vi "WS1050 Bench CAP Characterization_Ver1.3.vi"() -> ()   [LabVIEW 2012]
panel:
  in  "Cmd Full":string[](array[string])=["00", "01", "02", "03", "04", "05", "06", "07", "08", "09", "0A", "0B", "0C", "0D", "0E", "0F", "10", "11", "12", "13", "14", "15", "16", "17", "18", "19", "1A", "1B", "1C", "1D", "1E", "1F", "20", "21", "22", "23", "24", "25", "26", "27", "28", "29", "2A", "2B", "2C", "2D", "2E", "2F", "30", "31", "32", "33", "34", "35", "36", "37", "38", "39", "3A", "3B", "3A", "39", "38", "37", "36", "35", "34", "33", "32", "31", "30", "2F", "2E", "2D", "2C", "2B", "2A", "29", "28", "27", "26", "25", "24", "23", "22", "21", "20", "1F", "1E", "1D", "1C", "1B", "1A", "19", "18", "17", "16", "15", "14", "13", "12", "11", "10", "0F", "0E", "0D", "0C", "0B", "0A", "09", "08", "07", "06", "05", "04", "03", "02", "01", "00"]
  in  "Driver Name Full":string[](array[string])=["C1_Min", "F1_UP", "F2_UP", "F12_UP", "S1_UP", "S1F1_UP", "S1F2_UP", "S1F12_UP", "S2_UP", "S2F1_UP", "S2F2_UP", "S2F12_UP", "S3_UP", "S3F1_UP", "S3F2_UP", "S3F12_UP", "S4_UP", "S4F1_UP", "S4F2_UP", "S4F12_UP", "S5_UP", "S5F1_UP", "S5F2_UP", "S5F12_UP", "S6_UP", "S6F1_UP", "S6F2_UP", "S6F12_UP", "S7_UP", "S7F1_UP", "S7F2_UP", "S7F12_UP", "S8_UP", "S8F1_UP", "S8F2_UP", "S8F12_UP", "S9_UP", "S9F1_UP", "S9F2_UP", "S9F12_UP", "S10_UP", "S10F1_UP", "S10F2_UP", "S10F12_UP", "S11_UP", "S11F1_UP", "S11F2_UP", "S11F12_UP", "S12_UP", "S12F1_UP", "S12F2_UP", "S12F12_UP", "S13_UP", "S13F1_UP", "S13F2_UP", "S13F12_UP", "S14_UP", "S14F1_UP", "S14F2_UP", "S14F12_UP", "S14F2_DN", "S14F1_DN", "S14_DN", "S13F12_DN", "S13F2_DN", "S13F1_DN", "S13_DN", "S12F12_DN", "S12F2_DN", "S12F1_DN", "S12_DN", "S11F12_DN", "S11F2_DN", "S11F1_DN", "S11_DN", "S10F12_DN", "S10F2_DN", "S10F1_DN", "S10_DN", "S9F12_DN", "S9F2_DN", "S9F1_DN", "S9_DN", "S8F12_DN", "S8F2_DN", "S8F1_DN", "S8_DN", "S7F12_DN", "S7F2_DN", "S7F1_DN", "S7_DN", "S6F12_DN", "S6F2_DN", "S6F1_DN", "S6_DN", "S5F12_DN", "S5F2_DN", "S5F1_DN", "S5_DN", "S4F12_DN", "S4F2_DN", "S4F1_DN", "S4_DN", "S3F12_DN", "S3F2_DN", "S3F1_DN", "S3_DN", "S2F12_DN", "S2F2_DN", "S2F1_DN", "S2_DN", "S1F12_DN", "S1F2_DN", "S1F1_DN", "S1_DN", "F12_DN", "F2_DN", "F1_DN", "ALL_OFF"]
  in  "Tab Control":enum32{"CONTROL", "INDICATION"}(tab)
  in  "RFFE Com Port":refnum<visa-resource-name>="COM3"
  in  "AD7747 Com Port":refnum<visa-resource-name>="COM1"
  in  "Init":bool=TRUE
  in  "Wafer":string="WS1050"
  in  "Lot":string="Toggle 7"
  in  "SN":string="01"
  in  "Temperature":string="RT"
  in  "Delay(ms)":u32=100
  in  "TMN DC\\CAP Data Log File Path":path=path "C:/Andy Tr/Temp"
  in  "String":string="WS1050 BENCH CAP CHARACTERIZATION Ver1.3"
  out "C3Cal (pF)":dbl=-4.9974111328125
  out "C1Cal (pF)":dbl=-4.5642919921875
  out "C2Cal (pF)":dbl=-4.9191376953125
  out "S_ValueC3(pF)":dbl=-4.9974111328125
  out "S_ValueC1(pF)":dbl=-4.5642919921875
  out "S_ValueC2(pF)":dbl=-4.9191376953125
  in  "Calib Socket":bool
  out "C1_Mesa(pF)":dbl
  out "C2_Mesa(pF)":dbl
  out "C3_Mesa(pF)":dbl
  in  "A364X_VDD":refnum<visa-resource-name>="GPIB1::6::INSTR"
  in  "IDD Limit":dbl=0.02 format="%.2p"
  in  "VDD":dbl=3.3
  in  "CP Setting":i32(ring) items=["CP OFF", "CP ON", "DVA OFF", "DVA ON", "ECAL OFF", "ECAL ON", "CP 40.25V", "CP 35V", "CP 38V", "CP 44V", "CP 50V", "CP 23.75V", "CP 25.25V", "CP 29.75V", "C1 ON", "C1 OFF", "C2 ON", "C2 OFF", "C3 ON", "C3 OFF"]
  in  "Send":bool
  in  "Init AD7747":bool
  in  "Keithley 2000":refnum<visa-resource-name>
  out "C_min(pF)":string[](array[string])
  out "C_Max":string[](array[string])
  out "C_Min2(pF)":string[](array[string])
  out "error out":errorcluster
  in  "error in (no error)":errorcluster
  in  "stop":bool
  in  "Abort":bool
  in  "Start Test":bool
  out "Running loop":i32
  in  "Set Cmax":string[](array[string])=["07413B", "07423B", "07433B"]
  out "CMin_Hex":string[](array[string])
  out "CMax_Hex":string[](array[string])
  out "CMin2 Hex":string[](array[string])
  # "Company:  WiSpry Inc\n198 Fairbanks Ste 198 Irvine\n\nCreated by:  Andy V Tran\nDate:  03/11/2015\nTP:  WS1050 Bench\nCAP Characterization"
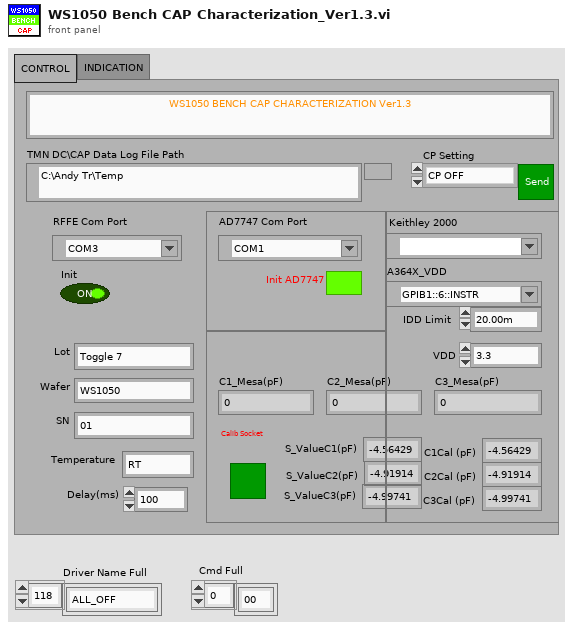
[diagram p1: front panel]
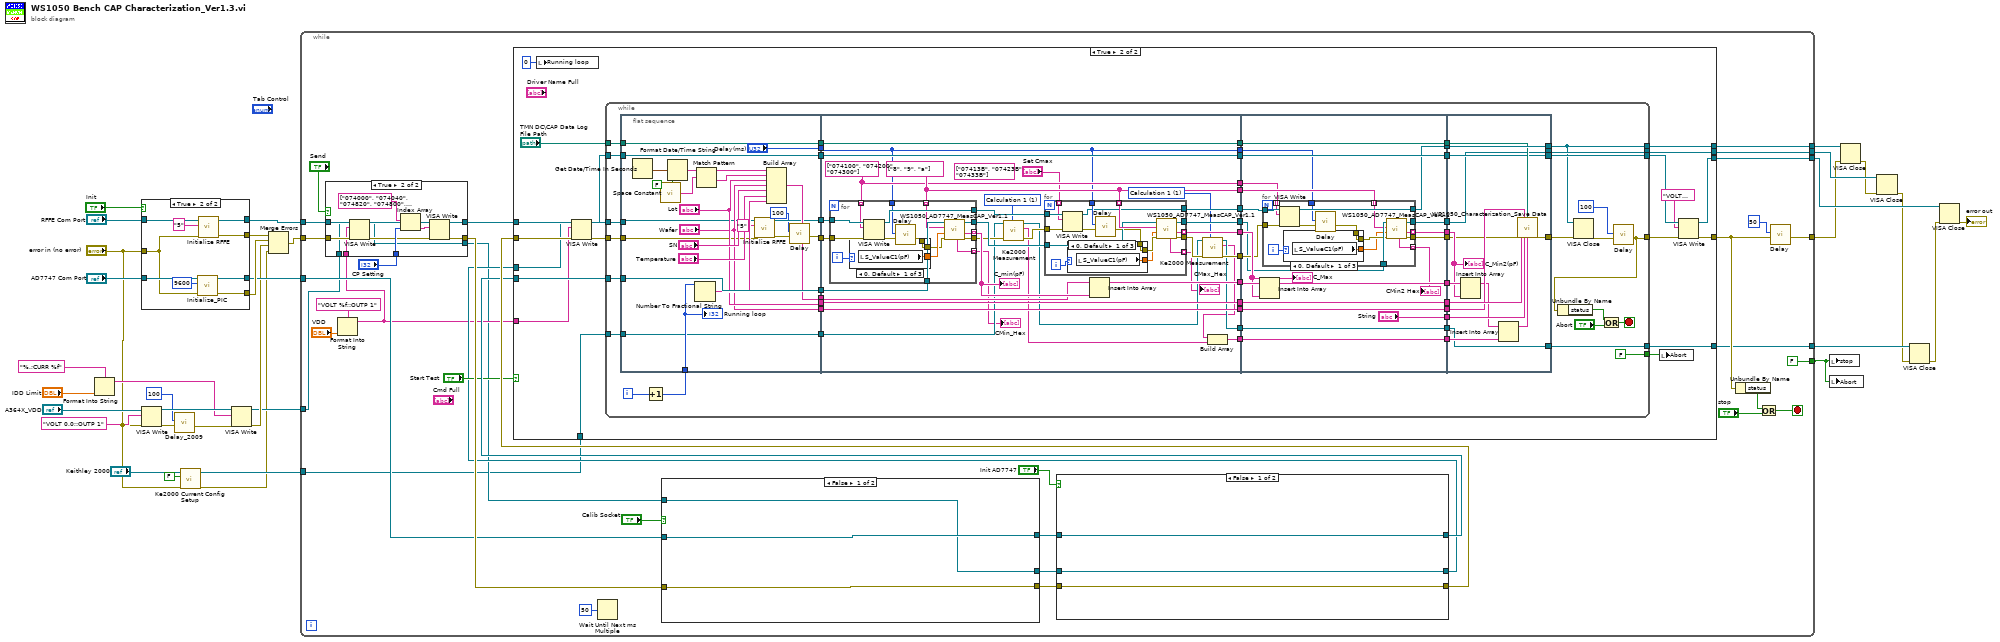
[diagram p0: block diagram]
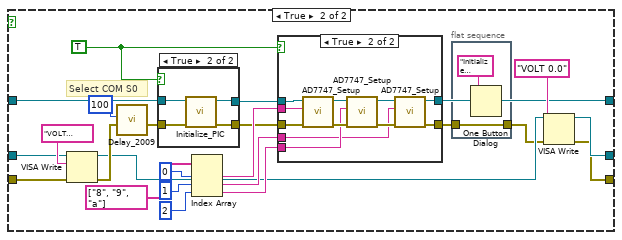
[diagram p3: hidden frame]
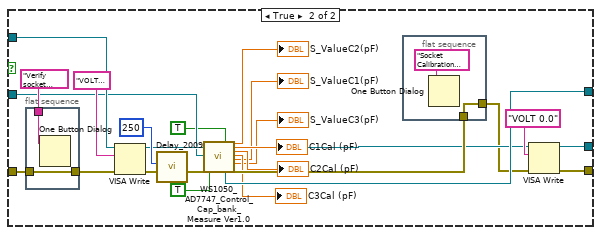
[diagram p6: hidden frame]
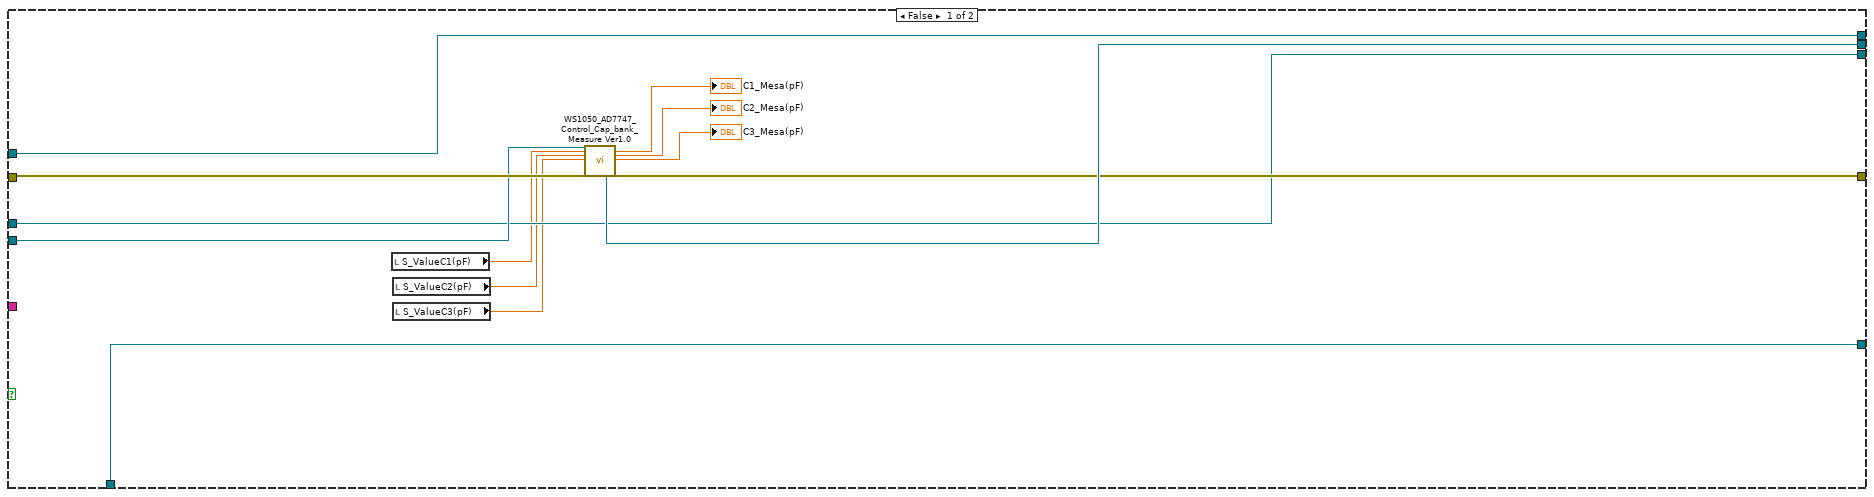
[diagram p7: hidden frame]
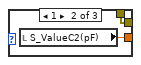
[diagram p8: hidden frame]
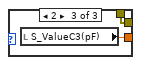
[diagram p9: hidden frame]
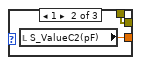
[diagram p10: hidden frame]
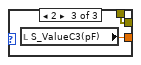
[diagram p11: hidden frame]
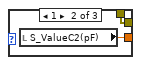
[diagram p12: hidden frame]
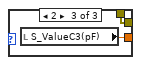
[diagram p13: hidden frame]
diagram:
  n1 = Format Into String(format string="%.;CURR %f", "IDD Limit") -> (resulting string=w24:string)  [unwired: 2 in, 1 out]
  n2 = case shown="True" "Init" {
    tunnel: "RFFE Com Port" -> [w37 w46]
    tunnel: [w37 w44] -> w33
    tunnel: "AD7747 Com Port" -> [w35 w42]
    tunnel: [w36 w41] -> w31
    tunnel: [w36 w40] -> w30
    tunnel: [w35 w39] -> w28
    tunnel: "error in (no error)" -> [w36 w38]
    frame False {
    }
    frame True {
      n3 = call "Initialize_PIC.vi"("error in (no error)"=w38, "baud rate"=u32 9600, "Select Com Port"=w42) -> ("error out"=w40:errorcluster, "VISA resource name out"=w39:refnum<visa-resource-name>)  [unwired: 7 in]
      n4 = call "Initialize RFFE.vi"("error in (no error)"=w38, "write buffer"="5", "Select Com Port"=w46) -> ("error out"=w41:errorcluster, "VISA resource name out"=w44:refnum<visa-resource-name>)  [unwired: 7 in]
    }
  }
  n5 = VISA Write(VISA resource name="A364X_VDD", write buffer="VOLT 0.0;:OUTP 1", error in (no error)="error in (no error)") -> (VISA resource name out=w25:refnum<visa-resource-name>, error out=w21:errorcluster)  [unwired: 1 out]
  n6 = call "Delay_2009.vi"("error in (no error)"=w21, "milliseconds to wait"=u32 100) -> ("error out"=w26:errorcluster)  [unwired: 9 in]
  n7 = call "Ke2000 Current Config Setup.vi"("error in (no error)"="error in (no error)", "Auto Range(T/F)"=FALSE, "VISA resource name"="Keithley 2000") -> ("error out"=w4:errorcluster, "VISA resource name out"=w5:refnum<visa-resource-name>)  [unwired: 7 in]
  n8 = VISA Write(VISA resource name=w25, write buffer=w24, error in (no error)=w26) -> (VISA resource name out=w16:refnum<visa-resource-name>, error out=w17:errorcluster)  [unwired: 1 out]
  n9 = Merge Errors(w31, w30, w17, w4) -> (w29:errorcluster)
  n10 = while {
    tunnel: w33 -> [w77]
    tunnel: w29 -> [w78]
    tunnel: w28 -> [w65]
    tunnel: [w73] -> w12
    tunnel: [w71] -> w15
    tunnel: [w70] -> w14
    tunnel: w16 -> [w52]
    tunnel: [w56] -> w13
    tunnel: [FALSE ("stop")] -> w9
    tunnel: w5 -> [w48]
    tunnel: [w47] -> w3
    stop <- w68 stop-if-true
    n11 = Format Into String(format string="VOLT %f;:OUTP 1", "VDD") -> (resulting string=w51:string)  [unwired: 2 in, 1 out]
    n12 = case shown="True" "Send" {
      tunnel: w78 -> [w410 w416]
      tunnel: [w410 w420] -> w66
      tunnel: [w409 w419] -> w76
      tunnel: "CP Setting" -> [_ w418]
      tunnel: w77 -> [w409 w417]
      tunnel: w52 -> [w408 w415]
      tunnel: w51 -> [_ w414]
      tunnel: [w408 w412] -> w50
      frame False {
      }
      frame True {
        n13 = VISA Write(VISA resource name=w415, write buffer=w414, error in (no error)=w416) -> (VISA resource name out=w412:refnum<visa-resource-name>, error out=w413:errorcluster)  [unwired: 1 out]
        n14 = Index Array(array=string[] ["074000", "074040", "074820", "074800", "074044", "074040", "074776", "07476F", "074773", "07477B", "07477C", "074760", "074762", "074768", "07413B", "074100", "07423B", "074200", "07433B", "074300"], index=w418) -> (element=w421:string)
        n15 = VISA Write(VISA resource name=w417, write buffer=w421, error in (no error)=w413) -> (VISA resource name out=w419:refnum<visa-resource-name>, error out=w420:errorcluster)  [unwired: 1 out]
      }
    }
    n16 = Wait Until Next ms Multiple(millisecond multiple=u32 50) -> ()  [unwired: 1 out]
    n17 = case shown="False" "Calib Socket" {
      tunnel: w66 -> [w131 w154]
      tunnel: [w131 w137] -> w60
      tunnel: w65 -> [w130 w135]
      tunnel: w50 -> [w129 w143]
      tunnel: [w129 w138] -> w61
      tunnel: [w130 w152] -> w59
      frame False {
      }
      frame True {
        n18 = flat-sequence {
          tunnel: [w157] -> w144
          tunnel: w154 -> [w157]
          tunnel: "Verify socket should be empty" ("message") -> [w156]
          frame #0 {
            n19 = One Button Dialog(message=w156) -> ()  [unwired: 1 in, 1 out]
          }
        }
        n20 = VISA Write(VISA resource name=w143, write buffer="VOLT 3.3;:OUTP 1", error in (no error)=w144) -> (VISA resource name out=w139:refnum<visa-resource-name>, error out=w141:errorcluster)  [unwired: 1 out]
        n21 = call "Delay_2009.vi"("error in (no error)"=w141, "milliseconds to wait"=u32 250) -> ("error out"=w134:errorcluster)  [unwired: 9 in]
        n22 = call "WS1050_AD7747_Control_Cap_bank_Measure Ver1.0.vi"("Select Com Port"=w135, "errorin"=w134, "Push Button to Measue Cap"=TRUE, "Push Button to Calibrate"=TRUE ("Push Button to Initialize AD7747")) -> ("Com Port Out"=w152:refnum<visa-resource-name>, "C2(pF)"=→"S_ValueC2(pF)":dbl, "C1_Mesa(pF)"=→"C1Cal (pF)":dbl, "C2_Mesa(pF)"=→"C2Cal (pF)":dbl, "C3_Mesa(pF)"=→"C3Cal (pF)":dbl, "C1(pF)"=→"S_ValueC1(pF)":dbl, "C3(pF)"=→"S_ValueC3(pF)":dbl, "error out"=w153:errorcluster)  [unwired: 16 in]
        n23 = flat-sequence {
          tunnel: [w158] -> w136
          tunnel: w153 -> [w158]
          frame #0 {
            n24 = One Button Dialog(message="Socket Calibration Completed, Please insert DUT into the Socket") -> ()  [unwired: 1 in, 1 out]
          }
        }
        n25 = VISA Write(VISA resource name=w139, write buffer="VOLT 0.0", error in (no error)=w136) -> (VISA resource name out=w138:refnum<visa-resource-name>, error out=w137:errorcluster)  [unwired: 1 out]
      }
    }
    n26 = case shown="False" "Init AD7747" {
      tunnel: w59 -> [w82 w107]
      tunnel: [w83 w87] -> w63
      tunnel: w60 -> [w83 w92]
      tunnel: [w82 w85] -> w62
      tunnel: w61 -> [w81 w93]
      tunnel: [w81 w88] -> w57
      frame False {
      }
      frame True {
        w97 = TRUE
        # "Select COM S0"
        n27 = VISA Write(VISA resource name=w93, write buffer="VOLT 3.3;:OUTP 1", error in (no error)=w92) -> (VISA resource name out=w89:refnum<visa-resource-name>, error out=w91:errorcluster)  [unwired: 1 out]
        n28 = call "Delay_2009.vi"("error in (no error)"=w91, "milliseconds to wait"=u32 100) -> ("error out"=w95:errorcluster)  [unwired: 9 in]
        n29 = case shown="True" w97 {
          tunnel: [w121 w126] -> w98
          tunnel: [w122 w125] -> w106
          tunnel: w107 -> [w122 w124]
          tunnel: w95 -> [w121 w123]
          frame False {
          }
          frame True {
            n30 = call "Initialize_PIC.vi"("error in (no error)"=w123, "Select Com Port"=w124) -> ("error out"=w126:errorcluster, "VISA resource name out"=w125:refnum<visa-resource-name>)  [unwired: 8 in]
          }
        }
        n31 = Index Array(array=string[] ["8", "9", "a"], index #1=0 ("index"), index #2=1 ("index"), index #3=2 ("index")) -> (element #1=w101:string, element #2=w100:string, element #3=w99:string)
        n32 = case shown="True" w97 {
          tunnel: w98 -> [w109 w112]
          tunnel: [w109 w110] -> w84
          tunnel: w106 -> [w108 w120]
          tunnel: w101 -> [_ w115]
          tunnel: w99 -> [_ w114]
          tunnel: w100 -> [_ w113]
          tunnel: [w108 w111] -> w85
          frame False {
          }
          frame True {
            n33 = call "AD7747_Setup.vi"("error in"=w112, "AD7747_Number"=w115, "Control"=w120) -> ("error out"=w119:errorcluster, "Control out"=w118:refnum<visa-resource-name>)  [unwired: 6 in, 1 out]
            n34 = call "AD7747_Setup.vi"("error in"=w119, "AD7747_Number"=w114, "Control"=w118) -> ("error out"=w117:errorcluster, "Control out"=w116:refnum<visa-resource-name>)  [unwired: 6 in, 1 out]
            n35 = call "AD7747_Setup.vi"("error in"=w117, "AD7747_Number"=w113, "Control"=w116) -> ("error out"=w110:errorcluster, "Control out"=w111:refnum<visa-resource-name>)  [unwired: 6 in, 1 out]
          }
        }
        n36 = flat-sequence {
          tunnel: w84 -> [w127]
          tunnel: [w127] -> w86
          frame #0 {
            n37 = One Button Dialog(message="Initialize AD7747 completed!") -> ()  [unwired: 1 in, 1 out]
          }
        }
        n38 = VISA Write(VISA resource name=w89, write buffer="VOLT 0.0", error in (no error)=w86) -> (VISA resource name out=w88:refnum<visa-resource-name>, error out=w87:errorcluster)  [unwired: 1 out]
      }
    }
    n39 = case shown="True" "Start Test" {
      tunnel: w76 -> [w165 w191]
      tunnel: w63 -> [w172 w186]
      tunnel: w62 -> [w171 w190]
      tunnel: [w169 w184] -> w74
      tunnel: [w165 w189] -> w71
      tunnel: [w170 w188] -> w70
      tunnel: w57 -> [w164 w185]
      tunnel: [w164 w181] -> w56
      tunnel: w51 -> [_ w176]
      tunnel: w48 -> [w160 w174]
      tunnel: [w160 w173] -> w47
      frame False {
        n40 = local read "S_ValueC1(pF)"() -> (w163:dbl)
        n41 = local read "S_ValueC2(pF)"() -> (w162:dbl)
        n42 = local read "S_ValueC3(pF)"() -> (w161:dbl)
        n43 = call "WS1050_AD7747_Control_Cap_bank_Measure Ver1.0.vi"("Select Com Port"=w171, "S_Value C1"=w163, "S_Value C2"=w162, "S_Value C3"=w161, "errorin"=w172) -> ("Com Port Out"=w170:refnum<visa-resource-name>, "C1_Mesa(pF)"=→"C1_Mesa(pF)":dbl, "C2_Mesa(pF)"=→"C2_Mesa(pF)":dbl, "C3_Mesa(pF)"=→"C3_Mesa(pF)":dbl, "error out"=w169:errorcluster)  [unwired: 15 in, 3 out]
      }
      frame True {
        n44 = local write "Running loop"(0 ("Loop Running")) -> ()
        n45 = VISA Write(VISA resource name=w185, write buffer=w176, error in (no error)=w186) -> (VISA resource name out=w183:refnum<visa-resource-name>, error out=w187:errorcluster)  [unwired: 1 out]
        n46 = while {
          tunnel: w191 -> [w244]
          tunnel: w187 -> [w243]
          tunnel: w190 -> [w242]
          tunnel: [w192] -> w180
          tunnel: "TMN DC\\CAP Data Log File Path" -> [w236]
          tunnel: [w202] -> w189
          tunnel: [w232] -> w188
          tunnel: w183 -> [w228]
          tunnel: [w225] -> w182
          tunnel: [FALSE ("Abort")] -> w177
          tunnel: w174 -> [w199]
          tunnel: [w193] -> w173
          i -> [w219]
          stop <- w239 stop-if-true
          n47 = flat-sequence {
            tunnel: w228 -> [w270]
            tunnel: w236 -> [w271]
            tunnel: w242 -> [w272]
            tunnel: w243 -> [w253]
            tunnel: w244 -> [w254]
            tunnel: [w250] -> w217
            tunnel: [w251] -> w216
            tunnel: [w272] -> w215
            tunnel: [w271] -> w214
            tunnel: [w270] -> w213
            tunnel: w212 -> [w257]
            tunnel: [w260] -> w211
            tunnel: ["Lot"] -> w210
            tunnel: ["Wafer"] -> w207
            tunnel: ["Delay(ms)"] -> w203
            tunnel: w199 -> [w248]
            tunnel: [w248] -> w198
            tunnel: [w295] -> w247
            tunnel: [w300] -> w246
            tunnel: [w282] -> w241
            tunnel: [w299] -> w235
            tunnel: [w298] -> w233
            tunnel: [w297] -> w230
            tunnel: [w294] -> w226
            tunnel: [w293] -> w224
            tunnel: [w288] -> w223
            tunnel: [w292] -> w222
            tunnel: w217 -> [w305]
            tunnel: w216 -> [w304]
            tunnel: w215 -> [w302]
            tunnel: w214 -> [w297]
            tunnel: w213 -> [w294]
            tunnel: w211 -> [w291]
            tunnel: w210 -> [w290]
            tunnel: [w290] -> w209
            tunnel: w207 -> [w289]
            tunnel: [w289] -> w206
            tunnel: w203 -> [w288]
            tunnel: w198 -> [w285]
            tunnel: [w280] -> w197
            tunnel: [w276] -> w195
            tunnel: w247 -> [w370]
            tunnel: w246 -> [w369]
            tunnel: [w368] -> w245
            tunnel: w241 -> [w364]
            tunnel: [w365] -> w240
            tunnel: w235 -> [w360]
            tunnel: [w359] -> w234
            tunnel: w233 -> [w358]
            tunnel: [w367] -> w231
            tunnel: w230 -> [w367]
            tunnel: [w366] -> w227
            tunnel: w226 -> [w366]
            tunnel: w224 -> [w363]
            tunnel: w223 -> [w362]
            tunnel: w222 -> [w361]
            tunnel: [w357] -> w221
            tunnel: [w356] -> w220
            tunnel: w209 -> [w355]
            tunnel: [w355] -> w208
            tunnel: w206 -> [w354]
            tunnel: [w354] -> w205
            tunnel: ["String"] -> w204
            tunnel: w197 -> [w352]
            tunnel: [w352] -> w196
            tunnel: w195 -> [w351]
            tunnel: [w351] -> w194
            tunnel: w245 -> [w402]
            tunnel: w240 -> [w397]
            tunnel: [w407] -> w201
            tunnel: w234 -> [w406]
            tunnel: [w406] -> w202
            tunnel: [w403] -> w232
            tunnel: w231 -> [w405]
            tunnel: w227 -> [w404]
            tunnel: [w404] -> w225
            tunnel: w221 -> [w403]
            tunnel: w220 -> [w401]
            tunnel: w208 -> [w400]
            tunnel: w205 -> [w399]
            tunnel: w204 -> [w398]
            tunnel: w196 -> [w393]
            tunnel: w194 -> [w395]
            tunnel: [w393] -> w193
            frame #0 {
              n48 = Get Date/Time In Seconds() -> (seconds since 1Jan1904=w266:timestamp)
              n49 = call <vilib>:"Space Constant.vi"() -> ("String"=w269:string)
              n50 = Format Date/Time String(seconds (now)=w266, UTC format=FALSE) -> (date/time string=w267:string)  [unwired: 1 out]
              n51 = Number To Fractional String(number=w257) -> (F-format string=w261:string)  [unwired: 3 in]
              n52 = Match Pattern(string=w267, regular expression=w269) -> (before substring=w265:string, after substring=w264:string)  [unwired: 3 out]
              n53 = call "Initialize RFFE.vi"("error in (no error)"=w253, "write buffer"="5", "Select Com Port"=w254) -> ("error out"=w252:errorcluster, "VISA resource name out"=w250:refnum<visa-resource-name>)  [unwired: 7 in]
              n54 = Build Array(w265, w264, "Lot", "Wafer", "SN", "Temperature", w261) -> (w260:string[])
              n55 = call "Delay.vi"("error in (no error)"=w252, "milliseconds to wait"=u32 100) -> ("error out"=w251:errorcluster)  [unwired: 9 in]
              "Running loop" <- w257
            }
            frame #1 {
              w279 = u16 1 items=["Function", "Calculation 1", "Calculation 2", "Calculation 3"] ("Source (0: Function)")
              w284 = u16 1 items=["Function", "Calculation 1", "Calculation 2", "Calculation 3"] ("Source (0: Function)")
              w293 = string[] ["8", "9", "a"]
              (unwired) string[] ["07413B", "07423B", "07433B"]
              w292 = string[] ["074100", "074200", "074300"]
              n56 = for {
                tunnel: w305 -> [w343]
                tunnel: w304 -> [w342]
                tunnel: w292 -> [w341] mode=indexing
                tunnel: [w340] -> w303
                tunnel: w302 -> [w339]
                tunnel: [w338] -> w301
                tunnel: [w337] -> w286
                tunnel: w288 -> [w335]
                tunnel: w293 -> [w334] mode=indexing
                tunnel: [w333] -> w296 mode=indexing
                tunnel: [w328] -> w274 mode=indexing
                i -> [w332]
                n57 = VISA Write(VISA resource name=w343, write buffer=w341, error in (no error)=w342) -> (VISA resource name out=w340:refnum<visa-resource-name>, error out=w336:errorcluster)  [unwired: 1 out]
                n58 = call "Delay.vi"("error in (no error)"=w336, "milliseconds to wait"=w335) -> ("error out"=w330:errorcluster)  [unwired: 9 in]
                n59 = case shown="0, Default" w332 {
                  tunnel: [w345 w347 w349] -> w331
                  tunnel: w330 -> [w344 w346 w348]
                  tunnel: [w344 w346 w348] -> w329
                  frame 0, Default {
                    n60 = local read "S_ValueC1(pF)"() -> (w345:dbl)
                  }
                  frame 1 {
                    n61 = local read "S_ValueC2(pF)"() -> (w347:dbl)
                  }
                  frame 2 {
                    n62 = local read "S_ValueC3(pF)"() -> (w349:dbl)
                  }
                }
                n63 = call "WS1050_AD7747_MeasCAP_Ver1.1.vi"("error in (no error)"=w329, "OFFSet Cal"=w331, "AD7747_Number"=w334, "Control"=w339) -> ("error"=w337:errorcluster, "CAP (pF)"=w333:string, "Control out"=w338:refnum<visa-resource-name>, "HEX"=w328:string)  [unwired: 3 in, 1 out]
              }
              "C_min(pF)" <- w296
              "CMin_Hex" <- w274
              n64 = call "Ke2000 Measurement.vi"("Source (0: Function)"=w284, "error in (no error)"=w286, "VISA resource name"=w285) -> ("error out"=w287:errorcluster, "Meas in micro"=w277:string, "VISA resource name out"=w281:refnum<visa-resource-name>)  [unwired: 3 in, 3 out]
              n65 = for {
                tunnel: w303 -> [w321]
                tunnel: w287 -> [w320]
                tunnel: "Set Cmax" -> [w319] mode=indexing
                tunnel: w288 -> [w317]
                tunnel: w293 -> [w316] mode=indexing
                tunnel: [w315] -> w283
                tunnel: [w314] -> w298
                tunnel: [w313] -> w299
                tunnel: w301 -> [w312]
                tunnel: [w311] -> w300 mode=indexing
                tunnel: [w306] -> w273 mode=indexing
                i -> [w309]
                n66 = VISA Write(VISA resource name=w321, write buffer=w319, error in (no error)=w320) -> (VISA resource name out=w313:refnum<visa-resource-name>, error out=w318:errorcluster)  [unwired: 1 out]
                n67 = call "Delay.vi"("error in (no error)"=w318, "milliseconds to wait"=w317) -> ("error out"=w308:errorcluster)  [unwired: 9 in]
                n68 = case shown="0, Default" w309 {
                  tunnel: [w323 w325 w327] -> w307
                  tunnel: w308 -> [w322 w324 w326]
                  tunnel: [w322 w324 w326] -> w310
                  frame 0, Default {
                    n69 = local read "S_ValueC1(pF)"() -> (w323:dbl)
                  }
                  frame 1 {
                    n70 = local read "S_ValueC2(pF)"() -> (w325:dbl)
                  }
                  frame 2 {
                    n71 = local read "S_ValueC3(pF)"() -> (w327:dbl)
                  }
                }
                n72 = call "WS1050_AD7747_MeasCAP_Ver1.1.vi"("error in (no error)"=w310, "OFFSet Cal"=w307, "AD7747_Number"=w316, "Control"=w312) -> ("error"=w315:errorcluster, "CAP (pF)"=w311:string, "Control out"=w314:refnum<visa-resource-name>, "HEX"=w306:string)  [unwired: 3 in, 1 out]
              }
              "CMax_Hex" <- w273
              n73 = Insert Into Array(array=w291, new element=w296) -> (w295:string[])  [unwired: 1 in]
              n74 = call "Ke2000 Measurement.vi"("Source (0: Function)"=w279, "error in (no error)"=w283, "VISA resource name"=w281) -> ("error out"=w282:errorcluster, "Meas in micro"=w278:string, "VISA resource name out"=w280:refnum<visa-resource-name>)  [unwired: 3 in, 3 out]
              n75 = Build Array(w278, w277) -> (w276:string[])
            }
            frame #2 {
              n76 = Insert Into Array(array=w370, new element=w369) -> (w368:string[])  [unwired: 1 in]
              n77 = for {
                tunnel: w360 -> [w386]
                tunnel: w364 -> [w385]
                tunnel: w361 -> [w384] mode=indexing
                tunnel: [w383] -> w359
                tunnel: w358 -> [w382]
                tunnel: [w381] -> w357
                tunnel: [w380] -> w365
                tunnel: w362 -> [w378]
                tunnel: w363 -> [w377] mode=indexing
                tunnel: [w376] -> w356 mode=indexing
                tunnel: [w371] -> w350 mode=indexing
                i -> [w375]
                n78 = VISA Write(VISA resource name=w386, write buffer=w384, error in (no error)=w385) -> (VISA resource name out=w383:refnum<visa-resource-name>, error out=w379:errorcluster)  [unwired: 1 out]
                n79 = call "Delay.vi"("error in (no error)"=w379, "milliseconds to wait"=w378) -> ("error out"=w373:errorcluster)  [unwired: 9 in]
                n80 = case shown="0, Default" w375 {
                  tunnel: [w388 w390 w392] -> w372
                  tunnel: w373 -> [w387 w389 w391]
                  tunnel: [w387 w389 w391] -> w374
                  frame 0, Default {
                    n81 = local read "S_ValueC1(pF)"() -> (w388:dbl)
                  }
                  frame 1 {
                    n82 = local read "S_ValueC2(pF)"() -> (w390:dbl)
                  }
                  frame 2 {
                    n83 = local read "S_ValueC3(pF)"() -> (w392:dbl)
                  }
                }
                n84 = call "WS1050_AD7747_MeasCAP_Ver1.1.vi"("error in (no error)"=w374, "OFFSet Cal"=w372, "AD7747_Number"=w377, "Control"=w382) -> ("error"=w380:errorcluster, "CAP (pF)"=w376:string, "Control out"=w381:refnum<visa-resource-name>, "HEX"=w371:string)  [unwired: 3 in, 1 out]
              }
              "CMin2 Hex" <- w350
              "C_Max" <- w369
            }
            frame #3 {
              n85 = Insert Into Array(array=w402, new element=w401) -> (w396:string[])  [unwired: 1 in]
              n86 = Insert Into Array(array=w396, new element=w395) -> (w394:string[])  [unwired: 1 in]
              n87 = call "WS1050_Characterization_Save Data.vi"("error in (no error)"=w397, "Lot"=w400, "Wafer"=w399, "TP"=w398, "TMN DC\\CAP Data Log File Path"=w405, "All Out"=w394) -> ("error out"=w407:errorcluster)  [unwired: 19 in, 2 out]
              "C_Min2(pF)" <- w401
            }
          }
          n88 = Increment(x=w219) -> (x+1=w212:i32)
          n89 = VISA Close(VISA resource name=w202, error in (no error)=w201) -> (error out=w200:errorcluster)
          n90 = call "Delay.vi"("error in (no error)"=w200, "milliseconds to wait"=u32 100) -> ("error out"=w192:errorcluster)  [unwired: 9 in]
          n91 = Unbundle By Name(w192) -> ("status"=w238:bool)
          n92 = Or(x=w238, y="Abort") -> (x .or. y?=w239:bool)
        }
        n93 = local write "Abort"(w177) -> ()
        n94 = VISA Write(VISA resource name=w182, write buffer="VOLT 0.0;:OUTP 0", error in (no error)=w180) -> (VISA resource name out=w181:refnum<visa-resource-name>, error out=w184:errorcluster)  [unwired: 1 out]
      }
    }
    n95 = Unbundle By Name(w74) -> ("status"=w75:bool)
    n96 = Or(x=w75, y="stop") -> (x .or. y?=w68:bool)
    n97 = call "Delay.vi"("error in (no error)"=w74, "milliseconds to wait"=u32 50) -> ("error out"=w73:errorcluster)  [unwired: 9 in]
  }
  n98 = local write "stop"(w9) -> ()
  n99 = local write "Abort"(w9) -> ()
  n100 = VISA Close(VISA resource name=w15, error in (no error)=w12) -> (error out=w11:errorcluster)
  n101 = VISA Close(VISA resource name=w14, error in (no error)=w11) -> (error out=w2:errorcluster)
  n102 = VISA Close(VISA resource name=w3, error in (no error)=w2) -> (error out=w1:errorcluster)
  n103 = VISA Close(VISA resource name=w13, error in (no error)=w1) -> (error out=→"error out":errorcluster)
